vi "DIO-432 and DIO-433 Write Protected Lines PointByPoint with Circuit Breaker - 3 channel.vi"() -> ()   [LabVIEW 8.6]
uses:
  <vilib>/UeiDaq/UeiDaqConfigureTimingForSimpleIO.vi
  <vilib>/UeiDaq/UeiDaqWriteOneDigitalScanUInt32.vi
  <vilib>/UeiDaq/UeiDaqWriteOneDigitalScanUInt16.vi
  <vilib>/UeiDaq/UeiDaqCreateAISession.vi
  <vilib>/UeiDaq/UeiDaqReadOneScaledScan.vi
  <vilib>/UeiDaq/UeiDaqCreateDOProtectedSession.vi
  <libdir>/resource/objmgr/UeiDaq.rc
panel:
  in  "ch2":bool
  in  "ch1":bool
  in  "ch0":bool caption="CB channel to reset"
  in  "PWM duty cycle ( 0 to 1 )":dbl[](array[numeric])
  in  "PWM period ( usec )":i32[](array[numeric])
  in  "Soft-start/stop length ( 256-5e6 usec )":i32[](array[numeric])
  in  "PWM mode":i32[](array[ring]) items=["Disables", "Soft-Start", "Soft-Stop", "Soft-start-stop", "Continuous", "Gated"]
  in  "Over/under count":i32
  out "CB status (lit if tripped)":bool[](array[boolean]) caption="Circuit breaker status (litted if tripped)"
  in  "CB reset and reenable":bool
  in  "Output line limits":cluster{"Line":i32, "Over-current ":dbl}[](array[cluster])
  out "Current measured at each output line":dbl[](array[numeric]) format="%.6f"
  in  "AI Resource (Guardian)":string
  in  "Auto-retry rate ( Hz )":dbl format="%.2f"
  in  "Auto-retry?":bool
  in  "Current measurement rate ( Hz )":dbl format="%.2f"
  out "raw data":u32[](array[numeric]) format="%x"
  out "current time":timestamp format="%<%X\n%x>T"
  out "# of DO ports":u32
  out "device name":string
  out "Do Resolution (bits)":u32
  in  "Digital Ports":bool[][](array[boolean])
  in  "DO Resource format string":string
  out "Total scans":u32
  in  "stop":bool
  # "DIO-432  and DIO-433 WRITE TO DIGITAL LINES (Point by Point) with CIRCUIT BREAKER"
  # "This program was created to demonstrate writing to 3 outputs \nwhile displaying self-testing guardian features, PMW control, and \ncircuit breaker features of the DIO-432/433."
  # "1/ Set the resource name -->"
  # "This example uses the \"doline\" syntax in \nthe DO resource string to separately configure\noutput lines."
  # "( 0-31 )"
  # "time dependant on measurement rate"
  # "Soft-start/stop length can be no longer than 255*period"
  # "Period determines transition rates of soft-start/stop length"
  # "Duty cylcle only altered during continuous and gated modes"
  # "2/ Set DO lines here - DO will be updated whenever a change is detected -->"
  # "ch0   ch1  ch2"
  # "digital I/O"
  # "600 mA limit per channel"
  # "device info"
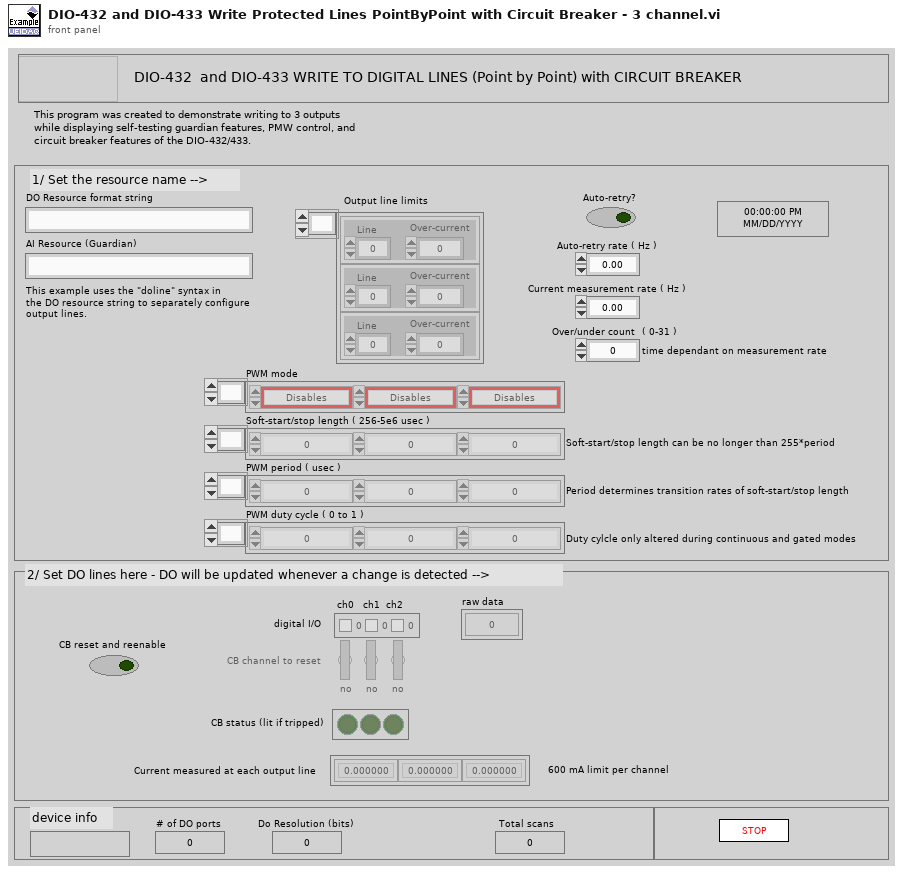
[diagram p1: front panel]
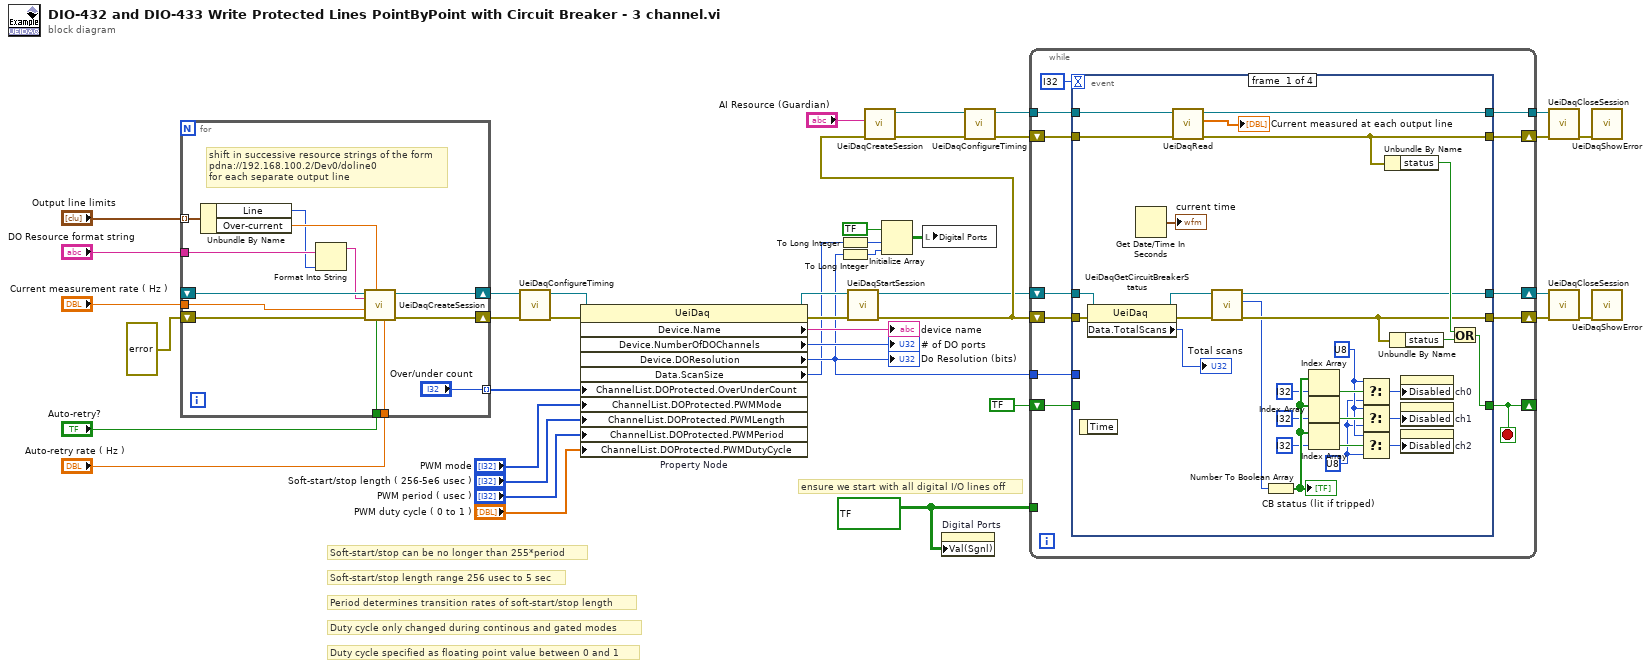
[diagram p0: block diagram]
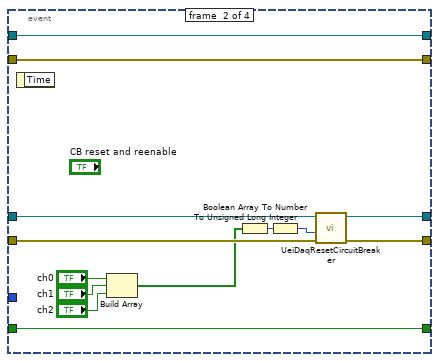
[diagram p2: hidden frame]
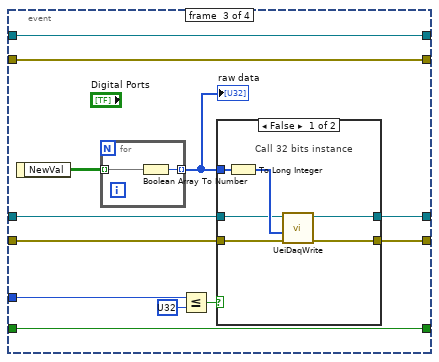
[diagram p3: hidden frame]
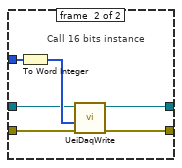
[diagram p4: hidden frame]
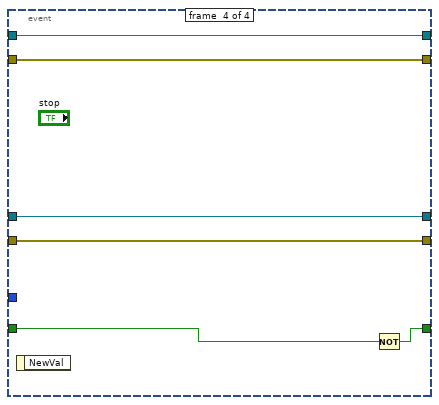
[diagram p5: hidden frame]
diagram:
  w2 = bool[][] ? ("Digital Ports")
  # "Duty cycle specified as floating point value between 0 and 1"
  # "Period determines transition rates of soft-start/stop length"
  # "Duty cycle only changed during continous and gated modes"
  # "Soft-start/stop length range 256 usec to 5 sec"
  # "Soft-start/stop can be no longer than 255*period"
  # "ensure we start with all digital I/O lines off"
  n1 = for {
    tunnel: "Current measurement rate ( Hz )" -> [w51]
    tunnel: "Auto-retry?" -> [w50]
    tunnel: "Auto-retry rate ( Hz )" -> [w49]
    shift-right: [w52] -> w38
    shift-left: errorcluster ? ("error out") -> [w48]
    shift-right: [w53] -> w39
    shift-left: _ -> [w47]
    tunnel: "DO Resource format string" -> [w45]
    tunnel: ["Over/under count"] -> w16 mode=indexing
    tunnel: "Output line limits" -> [w41] mode=indexing
    # "shift in successive resource strings of the form\npdna://192.168.100.2/Dev0/doline0 \nfor each separate output line"
    n2 = Unbundle By Name(w41) -> ("Line"=w44:i32, "Over-current"=w46:dbl)
    n3 = Format Into String(format string=w45, w44) -> (resulting string=w43:string)  [unwired: 2 in, 1 out]
    n4 = call-poly <vilib>:"UeiDaqCreateSession.vi"("Auto-retry rate"=w49, "Auto-retry?"=w50, "Over-current limit"=w46, "error in (no error)"=w48, "Current measurement rate"=w51, "Resource"=w43, "UeiDaq Refnum In"=w47) -> ("error out"=w52:errorcluster, "UeiDaq Refnum Out"=w53:refnum<k20>)  [unwired: 1 in, 2 out]
  }
  n5 = call-poly <vilib>:"UeiDaqConfigureTiming.vi"("error in (no error)"=w38, "UeiDaq Refnum In"=w39) -> ("error out"=w36:errorcluster, "UeiDaq Refnum Out"=w37:refnum<k20>)  [unwired: 1 in, 7 out]
  n6 = property on="Property Node" class="UeiDaq"(reference=w37, error in=w36, "ChannelList.DOProtected.OverUnderCount"=w16, "ChannelList.DOProtected.PWMMode"="PWM mode", "ChannelList.DOProtected.PWMLength"="Soft-start/stop length ( 256-5e6 usec )", "ChannelList.DOProtected.PWMPeriod"="PWM period ( usec )", "ChannelList.DOProtected.PWMDutyCycle"="PWM duty cycle ( 0 to 1 )") -> (reference out=w19:refnum<k20>, error out=w21:errorcluster, "Device.Name"=→"device name":string, "Device.NumberOfDOChannels"=→"# of DO ports":u32, "Device.DOResolution"=w10:u32, "Data.ScanSize"=w9:u32)
  "Do Resolution (bits)" <- w10
  n7 = To Long Integer(number=w9) -> (32bit integer=w12:i32)
  n8 = To Long Integer(number=w10) -> (32bit integer=w11:i32)
  n9 = call <vilib>:"UeiDaqStartSession.vi"("error in (no error)"=w21, "UeiDaq Refnum In"=w19) -> ("error out"=w20:errorcluster, "UeiDaq Refnum Out"=w18:refnum<k20>)  [unwired: 8 out]
  n10 = call-poly <vilib>:"UeiDaqCreateSession.vi"("error in (no error)"=w20, "Resource"="AI Resource (Guardian)") -> ("error out"=w26:errorcluster, "UeiDaq Refnum Out"=w27:refnum<k20>)  [unwired: 4 in, 4 out]
  n11 = Initialize Array(bool ? ("Boolean"), w12, w11) -> (w32:bool[][])
  n12 = local write "Digital Ports"(w32) -> ()
  n13 = property on="Digital Ports" class="Arr (strict)"("Val(Sgnl)"=w2) -> ()  [unwired: 2 in, 2 out]
  n14 = call-poly <vilib>:"UeiDaqConfigureTiming.vi"("error in (no error)"=w26, "UeiDaq Refnum In"=w27) -> ("error out"=w24:errorcluster, "UeiDaq Refnum Out"=w25:refnum<k20>)  [unwired: 1 in, 7 out]
  n15 = while {
    tunnel: w10 -> [w64]
    shift-right: [w62] -> w7
    shift-left: w20 -> [w63]
    shift-right: [w60] -> w8
    shift-left: w18 -> [w61]
    shift-right: [w58] -> _
    shift-left: bool ? ("x") -> [w59]
    tunnel: w25 -> [w57]
    tunnel: [w54] -> w22
    shift-right: [w55] -> w23
    shift-left: w24 -> [w56]
    tunnel: w2 -> [_]
    stop <- w58 stop-if-true
    n16 = event shown="[1] \"CB reset and reenable\": Value Change" {
      selector: _ -> [_ _ _ _]
      dyn-events: _ -> [_ _ _ _]
      timeout: i32 ? -> [_ _ _ _]
      tunnel: w63 -> [w94 w104 w117 w139]
      tunnel: w64 -> [_ _ w119 _]
      tunnel: [w81 w102 w113 w139] -> w62
      tunnel: w61 -> [w93 w105 w110 w138]
      tunnel: [w79 w103 w112 w138] -> w60
      tunnel: w59 -> [_ w101 w111 w137]
      tunnel: [w87 w101 w111 w136] -> w58
      tunnel: w57 -> [w90 w107 w109 w135]
      tunnel: w56 -> [w89 w106 w108 w134]
      tunnel: [w84 w106 w108 w134] -> w55
      tunnel: [w83 w107 w109 w135] -> w54
      event #0 {
        w72 = u8 ?
        w73 = u8 ?
        n17 = event-data() -> ()  [unwired: 2 out]
        n18 = property class="UeiDaq"(reference=w93, error in=w94) -> (reference out=w80:refnum<k20>, error out=w82:errorcluster, "Data.TotalScans"=→"Total scans":u32)
        n19 = Get Date/Time In Seconds() -> (seconds since 1Jan1904=→"current time":timestamp)
        n20 = call-poly <vilib>:"UeiDaqRead.vi"("error in (no error)"=w89, "UeiDaq Refnum In"=w90) -> ("error out"=w84:errorcluster, "Scaled Data"=→"Current measured at each output line":dbl[], "UeiDaq Refnum Out"=w83:refnum<k20>)  [unwired: 7 out]
        n21 = call <vilib>:"UeiDaqGetCircuitBreakerStatus.vi"("error in (no error)"=w82, "UeiDaq Refnum In"=w80) -> ("error out"=w81:errorcluster, "Current Status Mask"=w78:u32, "UeiDaq Refnum Out"=w79:refnum<k20>)  [unwired: 7 out]
        n22 = Number To Boolean Array(number=w78) -> (Boolean array=w77:bool[])
        "CB status (lit if tripped)" <- w77
        n23 = Index Array(array=w77, index=i32 ?) -> (element=w76:bool)
        n24 = Index Array(array=w77, index=i32 ?) -> (element=w74:bool)
        n25 = Index Array(array=w77, index=i32 ?) -> (element=w75:bool)
        n26 = Select(t=w73, s=w76, f=w72) -> (s? t:f=w71:u8)
        n27 = Select(t=w73, s=w74, f=w72) -> (s? t:f=w70:u8)
        n28 = Select(t=w73, s=w75, f=w72) -> (s? t:f=w69:u8)
        n29 = Unbundle By Name(w84) -> ("status"=w85:bool)
        n30 = Unbundle By Name(w81) -> ("status"=w86:bool)
        n31 = property on="ch0" class="Bool (strict)"("Disabled"=w71) -> ()  [unwired: 2 in, 2 out]
        n32 = property on="ch1" class="Bool (strict)"("Disabled"=w70) -> ()  [unwired: 2 in, 2 out]
        n33 = property on="ch2" class="Bool (strict)"("Disabled"=w69) -> ()  [unwired: 2 in, 2 out]
        n34 = Or(x=w85, y=w86) -> (x .or. y?=w87:bool)
      }
      event #1 {
        n35 = event-data() -> ()  [unwired: 2 out]
        n36 = Build Array("ch0", "ch1", "ch2") -> (w95:bool[])
        n37 = Boolean Array To Number(Boolean array=w95) -> (number=w100:u32)
        n38 = To Unsigned Long Integer(number=w100) -> (unsigned 32bit integer=w99:u32)
        n39 = call <vilib>:"UeiDaqResetCircuitBreaker.vi"("error in (no error)"=w104, "Reset Mask"=w99, "UeiDaq Refnum In"=w105) -> ("error out"=w102:errorcluster, "UeiDaq Refnum Out"=w103:refnum<k20>)  [unwired: 7 out]
      }
      event #2 {
        n40 = event-data() -> ("NewVal"=w115:bool[][])  [unwired: 1 out]
        n41 = for {
          tunnel: w115 -> [w132] mode=indexing
          tunnel: [w133] -> w114 mode=indexing
          n42 = Boolean Array To Number(Boolean array=w132) -> (number=w133:u32)
        }
        "raw data" <- w114
        n43 = Less Or Equal?(x=w119, y=u32 ?) -> (x <= y?=w116:bool)
        n44 = case shown="False" w116 {
          tunnel: w117 -> [w125 w131]
          tunnel: [w124 w130] -> w113
          tunnel: [w123 w129] -> w112
          tunnel: w114 -> [w122 w128]
          tunnel: w110 -> [w120 w126]
          frame #0 {
            # "Call 32 bits instance"
            n45 = To Long Integer(number=w122) -> (32bit integer=w121:i32[])
            n46 = call-poly <vilib>:"UeiDaqWrite.vi"("error in (no error)"=w125, "Digital Data"=w121, "UeiDaq Refnum In"=w120) -> ("error out"=w124:errorcluster, "UeiDaq Refnum Out"=w123:refnum<k20>)  [unwired: 7 out]
          }
          frame #1 {
            # "Call 16 bits instance"
            n47 = To Word Integer(number=w128) -> (16bit integer=w127:i16[])
            n48 = call-poly <vilib>:"UeiDaqWrite.vi"("error in (no error)"=w131, "Digital Data"=w127, "UeiDaq Refnum In"=w126) -> ("error out"=w130:errorcluster, "UeiDaq Refnum Out"=w129:refnum<k20>)  [unwired: 7 out]
          }
        }
      }
      event #3 {
        n49 = event-data() -> ()  [unwired: 2 out]
        n50 = Not(x=w137) -> (.not. x?=w136:bool)
      }
    }
  }
  n51 = call <vilib>:"UeiDaqCloseSession.vi"("error in (no error)"=w23, "UeiDaq Refnum In"=w22) -> ("error out"=w13:errorcluster)  [unwired: 1 in, 8 out]
  n52 = call <vilib>:"UeiDaqCloseSession.vi"("error in (no error)"=w7, "UeiDaq Refnum In"=w8) -> ("error out"=w40:errorcluster)  [unwired: 1 in, 8 out]
  n53 = call <vilib>:"UeiDaqShowError.vi"("error in (no error)"=w13) -> ()  [unwired: 1 in, 10 out]
  n54 = call <vilib>:"UeiDaqShowError.vi"("error in (no error)"=w40) -> ()  [unwired: 1 in, 10 out]
